vi "Build Interrupt Status Message.vi"(5 "State with Arguments":string, 7 "Arguments (\"\")":string) -> (6 "State with Arguments out":string)   [LabVIEW 2020, in "Communicable State Machine.lvlib"]
doc: "Builds a message that contains arguments for CSM. This VI will parse \"State with Arguments\" for message type, message string, arguments and target module from input <b>State with Arguments</b> and replace corresponding parts in the message with input values. The message type from input <b>State with Arguments</b> will be used.\n<B>For Example:</B>\nIf <b>State with Arguments</b> input is \"API: DoSth\"\nThen result string is \"API: DoSth >> Arguments\" as no message symbol is detected.\nIf <b>State with Arguments</b> input is \"API: DoSth >> Arguments -> Callee\"\nThen result string is \"API: DoSth >> NewArguments -> Callee\"\nIf <b>State with Arguments</b> input is \"API: DoSth >> Arguments -> Callee\"\nThen result string is \"API: DoSth >> NewArguments -> NewCallee\"\nIf <b>State with Arguments</b> input is \"API: DoSth >> Arguments -> Callee\"\nThen result string is \"API: DoSth -> NewCallee\"\nIf <b>State with Arguments</b> input is \"API: DoSth >> Arguments -@ Callee\"\nThen result string is \"API: DoSth >> NewArguments -@ Callee\"\n- <b>State with Arguments</b>: Input Message which might contain Arguments or target Module\n- <b>Arguments (\"\")</b>: The arguments which will be used to replace arguments in <b>State with Arguments</b>. if empty, no arguments will be included in output strings.\n- <b>Target Module (\"\")</b>: The target which will be used to replace target in <b>State with Arguments</b>. if empty, target in <b>State with Arguments</b> will be used.\n- <b>State with Arguments</b>: String stands for state with arguments\n\n<b>Inputs:</b>\n - <b>State with Arguments</b>:\n - <b>Arguments (\"\")</b>:\n\n<b>Outputs:</b>\n - <b>State with Arguments</b>:"
uses:
  Communicable State Machine.lvlib
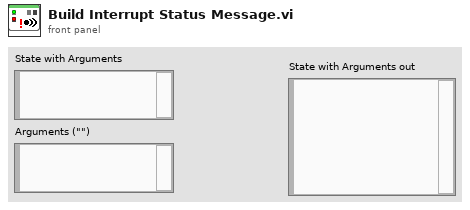
[diagram p1: front panel]
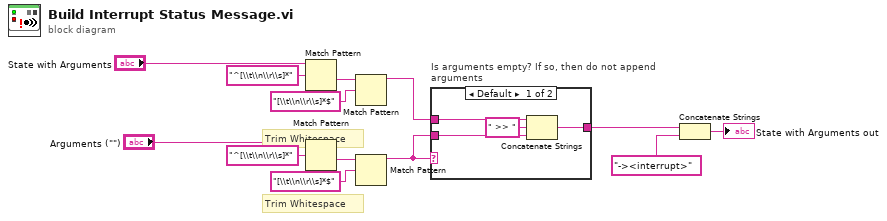
[diagram p0: block diagram]
diagram:
  # "Trim Whitespace"
  # "Trim Whitespace"
  n1 = Match Pattern(string="State with Arguments", regular expression="^[\\t\\n\\r\\s]*") -> (after substring=w6:string)  [unwired: 1 in, 3 out]
  n2 = Match Pattern(string="Arguments (\"\")", regular expression="^[\\t\\n\\r\\s]*") -> (after substring=w12:string)  [unwired: 1 in, 3 out]
  n3 = Match Pattern(string=w6, regular expression="[\\t\\n\\r\\s]*$") -> (before substring=w4:string)  [unwired: 1 in, 3 out]
  n4 = Match Pattern(string=w12, regular expression="[\\t\\n\\r\\s]*$") -> (before substring=w9:string)  [unwired: 1 in, 3 out]
  n5 = case "Is arguments empty? If so, then do not append arguments" shown="Default" w9 {
    tunnel: [w14 w18] -> w10
    tunnel: w4 -> [w17 w18]
    tunnel: w9 -> [w15 _]
    frame Default {
      n6 = Concatenate Strings(w17, " >> " ("string"), w15) -> (w14:string)
    }
    frame "" {
    }
  }
  n7 = Concatenate Strings(w10, "-><interrupt>" ("string")) -> (→"State with Arguments out":string)
